vi "02-sqrt_with_error_processing.vi"() -> ()   [LabVIEW 2018, in "LV2Julia_examples.lvlib"]
uses:
  LV2Julia_examples.lvlib
  LV2Julia_core/VIs/Server or client state.ctl
  LV2Julia_core/VIs/detailed error info.ctl
  LV2Julia_core/VIs/StackFrame.ctl
  LV2Julia_core/VIs/Commands.ctl
  71822543-7cbf-4033-aa74-7db116e85992.vi
  b897c894-e0b8-431a-8f01-351e2a203d12.vi
  58be0884-5f24-4db8-a231-ae1e3d7df6fe.vi
  <vilib>/Utility/High Resolution Relative Seconds.vi
  b897c894-e0b8-431a-8f01-351e2a203d12.vi/5e3eceae-b23b-45f8-ae21-4e9cd8df10ea.vi
  b897c894-e0b8-431a-8f01-351e2a203d12.vi/5e3eceae-b23b-45f8-ae21-4e9cd8df10ea.vi/161ab83e-e666-4cf8-90ca-a91b3d39a445.vi
  b897c894-e0b8-431a-8f01-351e2a203d12.vi/5e3eceae-b23b-45f8-ae21-4e9cd8df10ea.vi/3fec3670-9cc5-4d5c-8425-7c3dd7a75239.vi
  b897c894-e0b8-431a-8f01-351e2a203d12.vi/5e3eceae-b23b-45f8-ae21-4e9cd8df10ea.vi/31b8e5da-9b7a-4124-b3c5-22a32e8bf9ea.vi
  LV2Julia_core/VIs/jl-scripts path.vi
  LV2Julia_core/VIs/check ID validity.vi
  LV2Julia_core/VIs/bindata_descr to JSON.vi
  LV2Julia_core/VIs/check cluster field names.vi
  LV2Julia_core/VIs/concat JSON.vi
  LV2Julia_core/VIs/build request.vi
  LV2Julia_core/VIs/Parse server response.vi
  LV2Julia_core/VIs/log jl exceptions.vi
  LV2Julia_core/LV2Julia_core.lvlib
panel:
  out "call duration (ms)":dbl format="%#.2f"
  in  "x":dbl=2.0
  in  "next":bool
  out "sqrt":dbl=nan
  out "detailed error info":T1
  out "current error":errorcluster
  out "final error":errorcluster
  out "short err code":u8
  in  "stop":bool
  out "ZMQ timeout":bool
  out "Julia script file path":path
  out "temporary script path":path
  out "Jl Server state":T3
  # "On a negative argument, an exception occurs in Julia. \n\nThe Julia server catches the exception and passes the information to the LV client:  Below you get detailed error information. The Jula server keeps running and is ready to process the next request. Note that error processing in Julia can be slow.\n\nThe last 1024 (you can change the number) exceptions in the current session are logged into the global \"jl stack traces global.vi\".  On exception, this VI opens the front panel of that global."
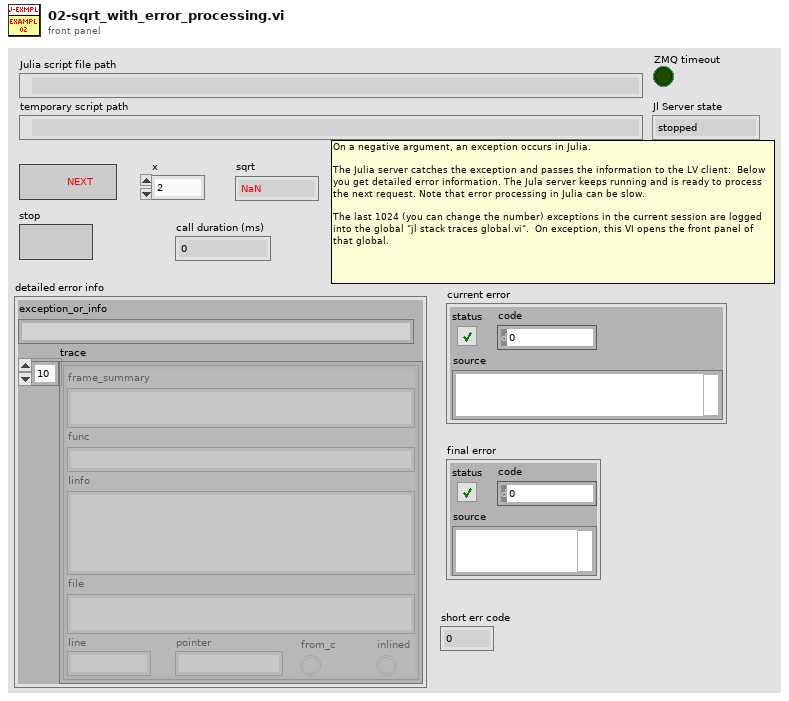
[diagram p1: front panel]
types:
  T1 = typedef "LV2Julia_core.lvlib/detailed error info.ctl" = cluster{"exception_or_info":string, "trace":T2[]}
  T2 = typedef "LV2Julia_core.lvlib/StackFrame.ctl" = cluster{"frame_summary":string, "func":string, "linfo":string, "file":string, "line":i32, "pointer":u64, "from_c":bool, "inlined":bool}
  T3 = typedef "LV2Julia_core.lvlib/Server or client state.ctl" = enum16{"stopped", "running", "unknown"}
  T4 = typedef "LV2Julia_core.lvlib/Commands.ctl" = enum16{"Start Jl-server & Init LV-client", "Send request & Get response ", "Stop Jl-server & Cleanup LV-client", "Cleanup LV-client", "Start Jl-server", "Stop Jl-server", "Init LV-Client", "Cleanup LV-Client", "(not allowed)", "Set LV Client state", "Set Jl Server state", "set ZMQ timeout", "read ZMQ timeout", "read-out state"}
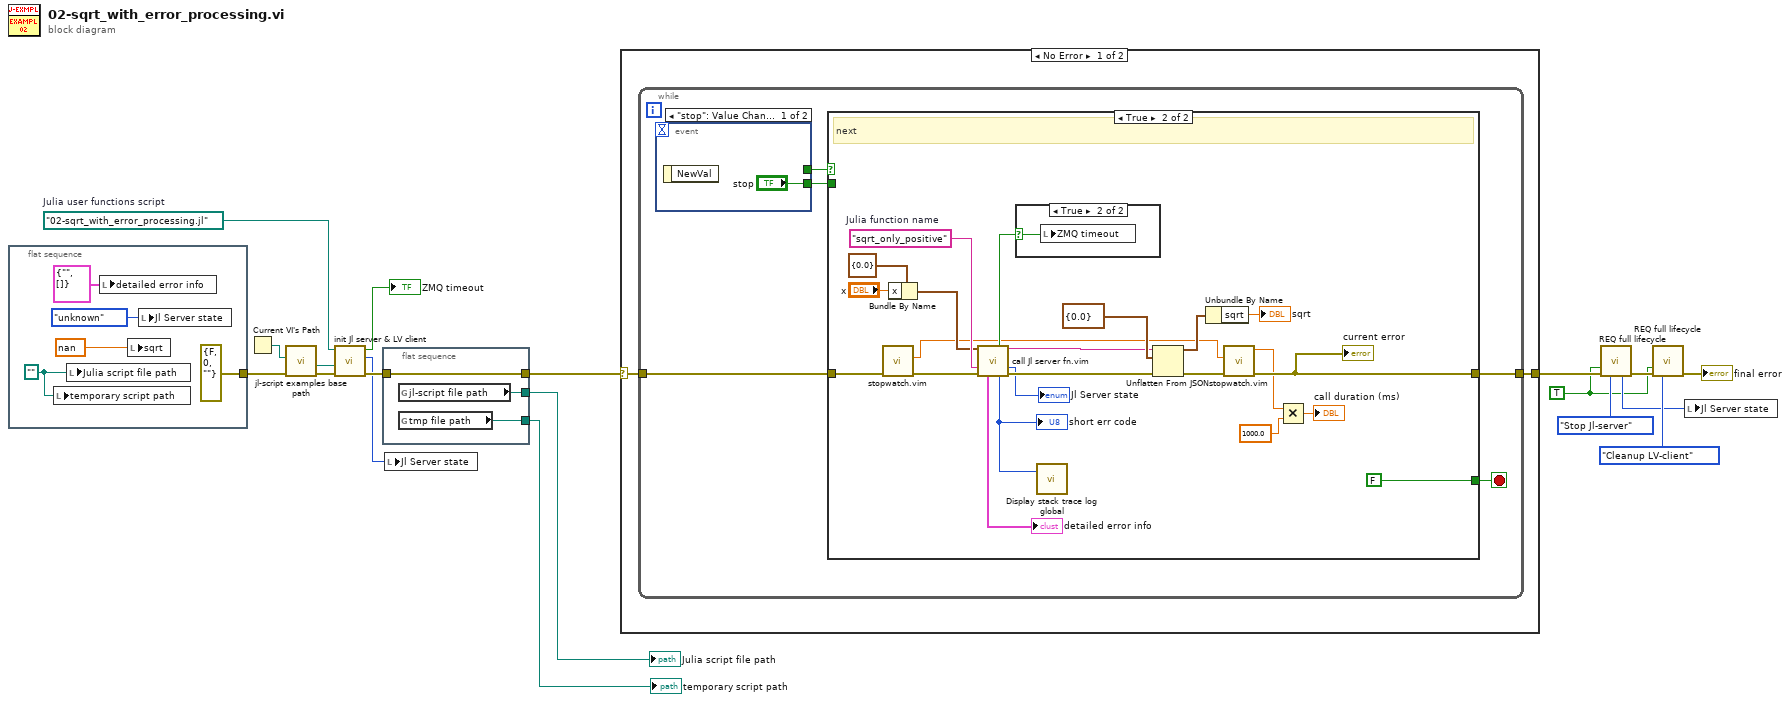
[diagram p0: block diagram]
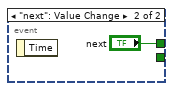
[diagram p2: hidden frame]
diagram:
  w8 = path "02-sqrt_with_error_processing.jl"  # Julia user functions script
  w9 = TRUE ("Force command")
  n1 = flat-sequence {
    tunnel: [errorcluster {"status"=FALSE, "code"=0, "source"=""} ("error in (no error)")] -> w3
    frame #0 {
      w19 = path ""
      n2 = local write "temporary script path"(w19) -> ()
      n3 = local write "Julia script file path"(w19) -> ()
      n4 = local write "detailed error info"(T1 {"exception_or_info"="", "trace"=[]} ("detailed error info")) -> ()
      n5 = local write "sqrt"(nan ("Server response")) -> ()
      n6 = local write "Jl Server state"(Server_or_client_state."unknown" ("Jl Server state out")) -> ()
    }
  }
  n7 = Current VI's Path() -> (path=w4:path)
  n8 = call "jl-script examples base path.vi"("error in (no error)"=w3, "calling example VI path"=w4) -> ("error out"=w2:errorcluster, "jl-script-examples base path"=w1:path)  [unwired: 8 in]
  n9 = call "init Jl server & LV client.vi"("error in (no error)"=w2, "Base path (not a path)"=w1, "Julia user functions script"=w8) -> ("error out"=w7:errorcluster, "Jl Server state out"=w5:T3, "timeout?"=→"ZMQ timeout":bool)  [unwired: 6 in]
  n10 = flat-sequence {
    tunnel: [w26] -> w13
    tunnel: w7 -> [w26]
    tunnel: [w25] -> w11
    tunnel: [w24] -> w12
    frame #0 {
      n11 = global read "jl-scripts path.vi" "jl-script file path"() -> (w25:path)
      n12 = global read "jl-scripts path.vi" "tmp file path"() -> (w24:path)
    }
  }
  n13 = local write "Jl Server state"(w5) -> ()
  n14 = case shown="No Error" w13 {
    selector: w13 -> [w27 w61]
    tunnel: [w28 w61] -> w18
    frame No Error {
      n15 = while {
        tunnel: w27 -> [w32]
        tunnel: [w33] -> w28
        stop <- w30 stop-if-true
        n16 = event shown="[0] \"stop\": Value Change" {
          selector: _ -> [_ _]
          dyn-events: _ -> [_ _]
          timeout: _ -> [_ _]
          tunnel: [_ "next"] -> w31
          tunnel: ["stop" _] -> w29
          event "stop": Value Change {
            n17 = event-data() -> ()  [unwired: 1 in, 1 out]
          }
          event "next": Value Change {
            n18 = event-data() -> ()  [unwired: 1 in, 1 out]
          }
        }
        n19 = case shown="True" w31 {
          tunnel: [w37 w40] -> w33
          tunnel: w32 -> [w37 w43]
          tunnel: [w36 FALSE ("stop this VI only")] -> w30
          tunnel: w29 -> [w36 _]
          frame False {
            # "stop"
          }
          frame True {
            w52 = "sqrt_only_positive"  # Julia function name
            # "next"
            n20 = call "stopwatch.vim"("anything in"=w43) -> ("copy of anything out"=w42:errorcluster, "current timepoint"=w39:dbl)  [unwired: 8 in, 1 out]
            n21 = Bundle By Name(cluster=cluster{"x":dbl} {"x"=0.0}, "x"="x") -> (w51:cluster{"x":dbl})
            n22 = call "call Jl server fn.vim"("Arguments 1"=w51, "fun2call"=w52, "error in (no error)"=w42) -> ("timeout?"=w48:bool, "JSON received"=w47:string, "Jl Server state out"=→"Jl Server state":T3, "detailed error info"=→"detailed error info":T1, "return code"=w46:u8, "error out"=w53:errorcluster)  [unwired: 6 in, 1 out]
            "short err code" <- w46
            n23 = case shown="True" w48 {
              selector: w48 -> [_ w60]
              frame False {
              }
              frame True {
                n24 = local write "ZMQ timeout"(w60) -> ()
              }
            }
            n25 = call "Display stack trace log global.vi"("server return code"=w46) -> ()  [unwired: 3 in]
            n26 = Unflatten From JSON(JSON string=w47, type and defaults=cluster{"sqrt":dbl} {"sqrt"=0.0} ("parsed response"), error in (no error)=w53) -> (value=w58:cluster{"sqrt":dbl}, error out=w41:errorcluster)  [unwired: 4 in]
            n27 = Unbundle By Name(w58) -> ("sqrt"=→"sqrt":dbl)
            n28 = call "stopwatch.vim"("anything in"=w41, "prev timepoint (0)"=w39) -> ("copy of anything out"=w40:errorcluster, "delta t (s)"=w38:dbl)  [unwired: 7 in, 1 out]
            "current error" <- w40
            n29 = Multiply(x=w38, y=1000.0) -> (x*y=→"call duration (ms)":dbl)
          }
        }
      }
    }
    frame Error {
    }
  }
  n30 = call "REQ full lifecycle.vi"("Force command"=w9, "error in"=w18, "command"=Commands."Stop Jl-server") -> ("Jl Server state out"=w10:T3, "error out"=w16:errorcluster)  [unwired: 6 in, 5 out]
  n31 = call "REQ full lifecycle.vi"("Force command"=w9, "error in"=w16, "command"=Commands."Cleanup LV-client") -> ("error out"=→"final error":errorcluster)  [unwired: 6 in, 6 out]
  n32 = local write "Jl Server state"(w10) -> ()
  "temporary script path" <- w12
  "Julia script file path" <- w11
